vi "mediaRobos_v2.vi"(11 "Array Robot Pose + CamID":T1(array[cluster])) -> (3 "Array":cluster{"x":dbl, "y":dbl, "robot_id":i32}[](array[cluster]))   [LabVIEW 2018]
panel:
  in  "cluster":cluster{"x":dbl, "y":dbl, "robot_id":i32}
  in  "Field Size 2":T2
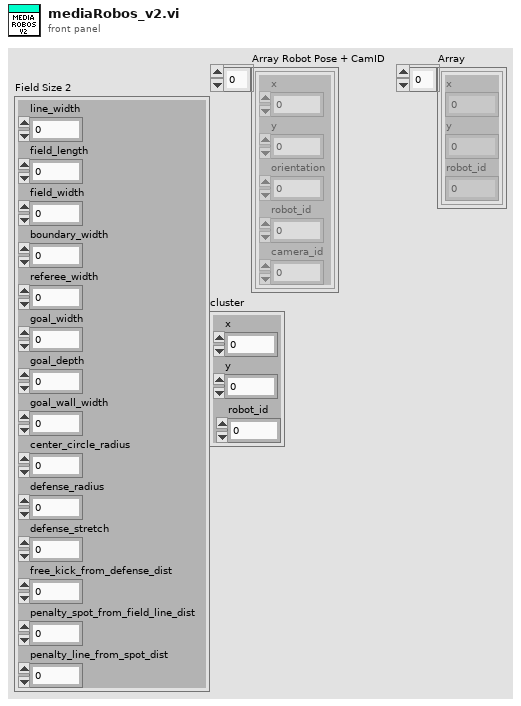
[diagram p1: front panel]
types:
  T1 = cluster{"x":sgl, "y":sgl, "orientation":sgl, "robot_id":u32, "camera_id":u32}[]
  T2 = cluster{"line_width":u32, "field_length":u32, "field_width":u32, "boundary_width":u32, "referee_width":u32, "goal_width":u32, "goal_depth":u32, "goal_wall_width":u32, "center_circle_radius":u32, "defense_radius":u32, "defense_stretch":u32, "free_kick_from_defense_dist":u32, "penalty_spot_from_field_line_dist":u32, "penalty_line_from_spot_dist":u32}
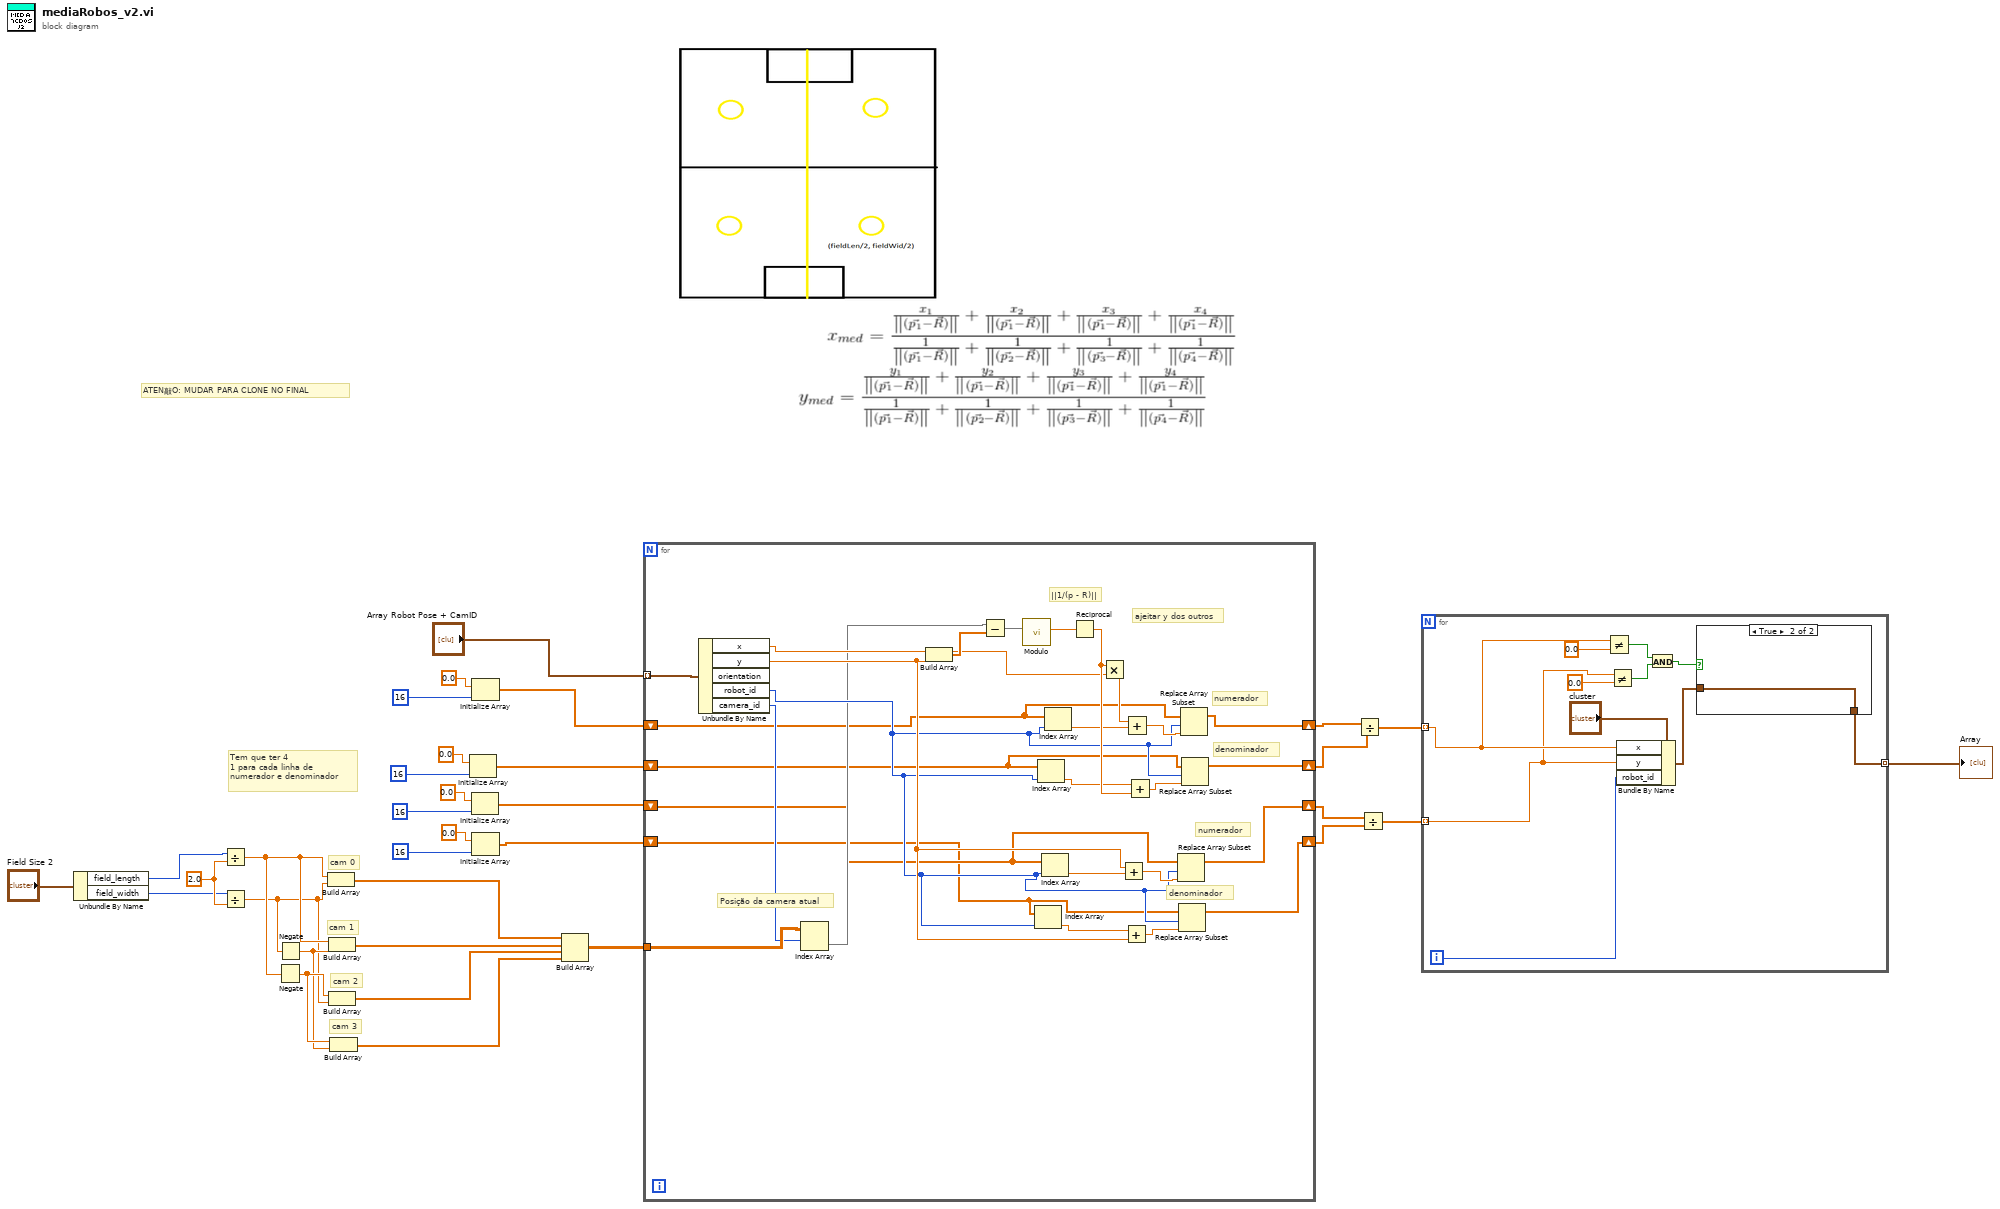
[diagram p0: block diagram]
diagram:
  w32 = 2.0 ("y")
  # "Tem que ter 4\n1 para cada linha de\nnumerador e denominador"
  # "cam 3"
  # "cam 2"
  # "cam 1"
  # "cam 0"
  # "ATEN敲O: MUDAR PARA CLONE NO FINAL"
  n1 = Unbundle By Name("Field Size 2") -> ("field_length"=w31:u32, "field_width"=w30:u32)
  n2 = Divide(x=w31, y=w32) -> (x/y=w28:dbl)
  n3 = Divide(x=w30, y=w32) -> (x/y=w26:dbl)
  n4 = Negate(x=w28) -> (-x=w29:dbl)
  n5 = Negate(x=w26) -> (-x=w27:dbl)
  n6 = Build Array(w28, w26) -> (w25:dbl[])
  n7 = Build Array(w28, w27) -> (w24:dbl[])
  n8 = Build Array(w29, w26) -> (w23:dbl[])
  n9 = Build Array(w29, w27) -> (w22:dbl[])
  n10 = Initialize Array(0.0 ("element"), 16 ("dimension size")) -> (w10:dbl[])
  n11 = Initialize Array(0.0 ("element"), 16 ("dimension size")) -> (w9:dbl[])
  n12 = Initialize Array(0.0 ("element"), 16 ("dimension size")) -> (w11:dbl[])
  n13 = Initialize Array(0.0 ("element"), 16 ("dimension size")) -> (w8:dbl[])
  n14 = Build Array(w25, w24, w23, w22) -> (w20:dbl[][])
  n15 = for {
    tunnel: "Array Robot Pose + CamID" -> [w61] mode=indexing
    tunnel: w20 -> [w60]
    shift-right: [w41] -> w7
    shift-left: w11 -> [w35]
    shift-right: [w40] -> w6
    shift-left: w10 -> [w34]
    shift-right: [w39] -> w5
    shift-left: w9 -> [w37]
    shift-right: [w38] -> w4
    shift-left: w8 -> [w36]
    # "ajeitar y dos outros"
    # "denominador"
    # "numerador"
    # "denominador"
    # "numerador"
    # "||1/(p - R)||"
    # "Posição da camera atual"
    n16 = Unbundle By Name(w61) -> ("x"=w49:sgl, "y"=w48:sgl, "robot_id"=w47:u32, "camera_id"=w59:u32)  [unwired: 1 out]
    n17 = Index Array(array=w60, index (row)=w59) -> (element=w46:dbl[])  [unwired: 1 in]
    n18 = Build Array(w49, w48) -> (w58:sgl[])
    n19 = Subtract(x=w46, y=w58) -> (x-y=w57:dbl[])
    n20 = call "Modulo.vi"("2D vector"=w57) -> ("Modulo"=w56:dbl)  [unwired: 10 in]
    n21 = Index Array(array=w36, index=w47) -> (element=w42:dbl)
    n22 = Index Array(array=w34, index=w47) -> (element=w44:dbl)
    n23 = Index Array(array=w37, index=w47) -> (element=w43:dbl)
    n24 = Index Array(array=w35, index=w47) -> (element=w45:dbl)
    n25 = Reciprocal(x=w56) -> (1/x=w50:dbl)
    n26 = Multiply(x=w50, y=w49) -> (x*y=w55:dbl)
    n27 = Add(x=w48, y=w43) -> (x+y=w52:dbl)
    n28 = Add(x=w42, y=w48) -> (x+y=w51:dbl)
    n29 = Add(x=w55, y=w45) -> (x+y=w54:dbl)
    n30 = Add(x=w44, y=w50) -> (x+y=w53:dbl)
    n31 = Replace Array Subset(array=w37, new element=w52, index=w47) -> (w39:dbl[])
    n32 = Replace Array Subset(array=w36, new element=w51, index=w47) -> (w38:dbl[])
    n33 = Replace Array Subset(array=w35, new element=w54, index=w47) -> (w41:dbl[])
    n34 = Replace Array Subset(array=w34, new element=w53, index=w47) -> (w40:dbl[])
  }
  n35 = Divide(x=w7, y=w6) -> (x/y=w3:dbl[])
  n36 = Divide(x=w5, y=w4) -> (x/y=w2:dbl[])
  n37 = for {
    tunnel: w3 -> [w71] mode=indexing
    tunnel: w2 -> [w68] mode=indexing
    tunnel: [w64] -> w1 mode=indexing
    i -> [w72]
    n38 = Not Equal?(x=w71, y=0.0) -> (x != y?=w67:bool)
    n39 = Not Equal?(x=w68, y=0.0) -> (x != y?=w66:bool)
    n40 = Bundle By Name(cluster="cluster", "x"=w71, "y"=w68, "robot_id"=w72) -> (w63:cluster{"x":dbl, "y":dbl, "robot_id":i32})
    n41 = And(x=w67, y=w66) -> (x .and. y?=w65:bool)
    n42 = case shown="True" w65 {
      tunnel: [w73 w74] -> w64
      tunnel: w63 -> [w73 w74]
      frame False {
      }
      frame True {
      }
    }
  }
  "Array" <- w1
